vi "Voltage_Transformation.vi"(10 "VLL":sgl[](array[numeric]) format="%#_13g") -> (2 "VLN":sgl[](array[numeric]))   [LabVIEW 2018]
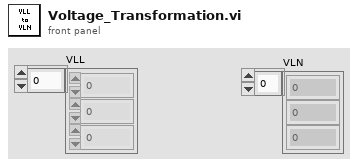
[diagram p1: front panel]
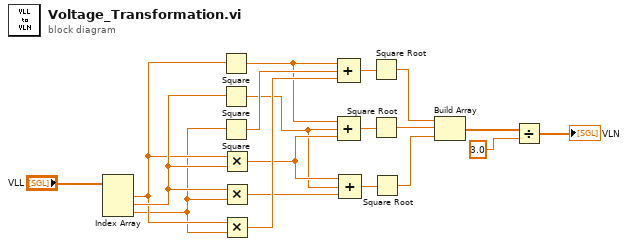
[diagram p0: block diagram]
diagram:
  n1 = Index Array(array="VLL") -> (element #1=w17:sgl, element #2=w18:sgl, element #3=w16:sgl)  [unwired: 3 in]
  n2 = Square(x=w17) -> (x^2=w10:sgl)
  n3 = Square(x=w18) -> (x^2=w7:sgl)
  n4 = Square(x=w16) -> (x^2=w12:sgl)
  n5 = Multiply(x=w17, y=w18) -> (x*y=w8:sgl)
  n6 = Multiply(x=w18, y=w16) -> (x*y=w9:sgl)
  n7 = Multiply(x=w17, y=w16) -> (x*y=w15:sgl)
  n8 = Compound Arithmetic op=ADD(w10, w12, w15) -> (w14:sgl)
  n9 = Compound Arithmetic op=ADD(w10, w7, w8) -> (w13:sgl)
  n10 = Compound Arithmetic op=ADD(w8, w7, w9) -> (w11:sgl)
  n11 = Square Root(x=w14) -> (sqrt(x)=w6:sgl)
  n12 = Square Root(x=w13) -> (sqrt(x)=w5:sgl)
  n13 = Square Root(x=w11) -> (sqrt(x)=w4:sgl)
  n14 = Build Array(w6, w5, w4) -> (w3:sgl[])
  n15 = Divide(x=w3, y=3.0) -> (x/y=→"VLN":dbl[])
